vi "UART Read Byte Array.vi"(8 "Error In":errorcluster, 9 "Num Bytes":u8, 10 "UART Channel (0)":u8, 11 "LINX Resource":T1) -> (0 "Error Out":errorcluster, 2 "Data":u8[](array[numeric]), 3 "LINX Resource":T1)   [LabVIEW 2014, in "LMH-LINX.lvlib"]
doc: "Read the specified number of bytes from the specified UART channel's receive buffer as a byte array."
uses:
  LMH-LINX.lvlib
  Private/Type Defs/LINX Ref.ctl
  Private/Type Defs/Platform.ctl
  Private/Type Defs/Interface.ctl
  Private/Device/Type Defs/LINX Device Config.ctl
  Private/Device/Type Defs/TCP Config.ctl
  Private/Device/Type Defs/Channels.ctl
  Private/Type Defs/Peripheral.ctl
  Private/Type Defs/Channel FGV States.ctl
  Private/Device/Device.lvlib
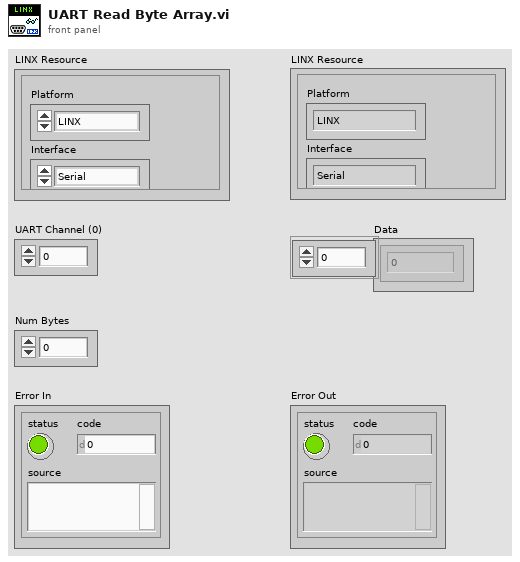
[diagram p1: front panel]
types:
  T1 = typedef "LMH-LINX.lvlib/LINX Ref.ctl" = cluster{"Platform":T2, "Interface":T3, "LINX Device Config":T4}
  T2 = typedef "LMH-LINX.lvlib/Platform.ctl" = enum16{"LINX", "myRIO"}
  T3 = typedef "LMH-LINX.lvlib/Interface.ctl" = enum16{"Serial", "TCP"}
  T4 = typedef "LMH-LINX.lvlib/Device.lvlib/LINX Device Config.ctl" = cluster{"Interface":T3, "COM Port":refnum<visa-resource-name>, "TCP Configuration":T5, "Device Family":u8, "Device ID":u8, "Device Name":string, "TCP Ref":refnum<k5>, "Channels":T6}
  T5 = typedef "LMH-LINX.lvlib/Device.lvlib/TCP Config.ctl" = cluster{"IP Address":string, "Port":u16}
  T6 = typedef "LMH-LINX.lvlib/Channels.ctl" = cluster{"DI":u8[], "DO":u8[], "AI":u8[], "AO":u8[], "PWM":u8[], "QE":u8[], "UART":u8[], "I2C 2":u8[], "SPI":u8[], "CAN":u8[], "Servo":u8[], "AI Ref (V)":dbl, "AO Ref (V)":dbl, "AO Resolution (Bits)":u8}
  T7 = typedef "LMH-LINX.lvlib/Peripheral.ctl" = enum8{"DI", "DO", "AI", "AO", "PWM", "QE", "UART", "I2C", "SPI", "CAN", "Servo"}
  T8 = typedef "LMH-LINX.lvlib/Channel FGV States.ctl" = enum16{"Initialize", "Get", "Set"}
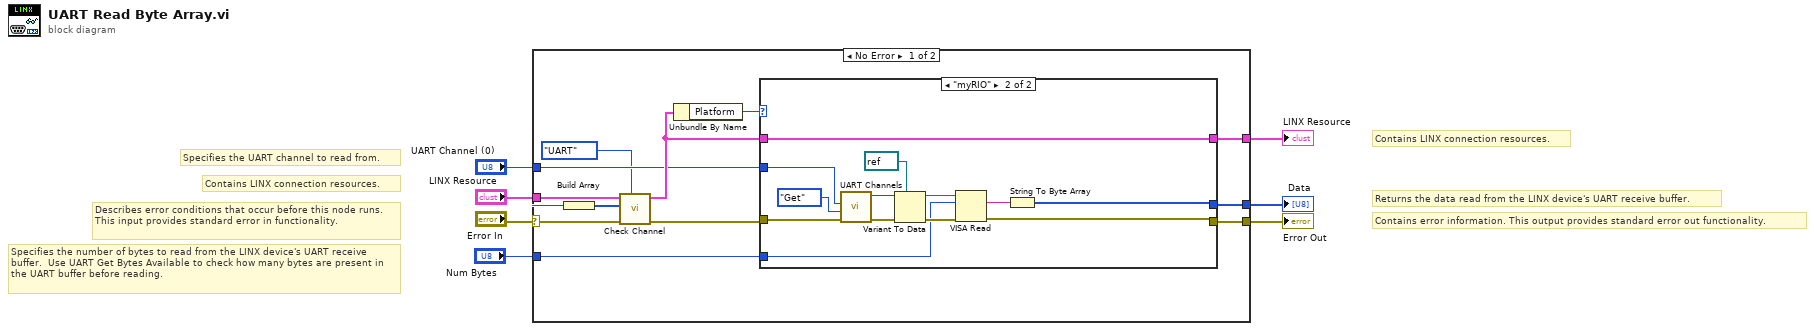
[diagram p0: block diagram]
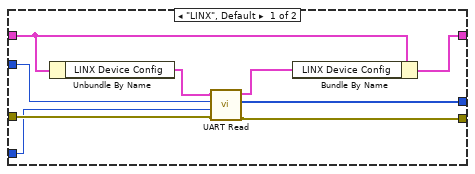
[diagram p2: hidden frame]
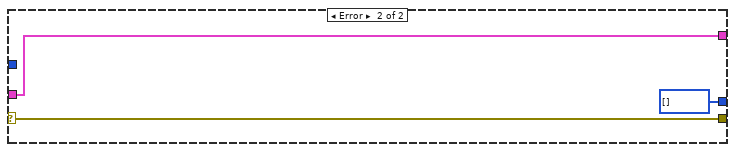
[diagram p3: hidden frame]
diagram:
  # "Specifies the number of bytes to read from the LINX device's UART receive buffer.  Use UART Get Bytes Available to check how many bytes are present in the UART buffer before reading."
  # "Specifies the UART channel to read from."
  # "Returns the data read from the LINX device's UART receive buffer."
  # "Contains LINX connection resources."
  # "Contains error information. This output provides standard error out functionality."
  # "Contains LINX connection resources."
  # "Describes error conditions that occur before this node runs. This input provides standard error in functionality."
  n1 = case shown="No Error" "Error In" {
    selector: "Error In" -> [w8 w44]
    tunnel: [w18 w44] -> w7
    tunnel: [w17 w43] -> w6
    tunnel: "LINX Resource" -> [w16 w43]
    tunnel: "UART Channel (0)" -> [w12 _]
    tunnel: "Num Bytes" -> [w10 _]
    tunnel: [w9 u8[] [] ("unsigned byte array")] -> w2
    frame No Error {
      n2 = Build Array(w12) -> (w13:u8[])
      n3 = call "Check Channel.vi"("Peripheral"=Peripheral."UART", "Error In"=w8, "Channels"=w13, "LINX Resource"=w16) -> ("Error Out"=w14:errorcluster, "LINX Resource"=w15:T1)  [unwired: 5 in, 1 out]
      n4 = Unbundle By Name(w15) -> ("Platform"=w19:T2)
      n5 = case shown="\"myRIO\"" w19 {
        tunnel: w14 -> [w25 w40]
        tunnel: w15 -> [w28 w41]
        tunnel: [w26 w32] -> w18
        tunnel: [w27 w41] -> w17
        tunnel: w12 -> [w21 w36]
        tunnel: [w22 w29] -> w9
        tunnel: w10 -> [w20 w31]
        frame "LINX", Default {
          n6 = Unbundle By Name(w28) -> ("LINX Device Config"=w24:T4)
          n7 = call "UART Read.vi"("Error In"=w25, "Num Bytes"=w20, "UART Channel"=w21, "LINX Device Config"=w24) -> ("Error Out"=w26:errorcluster, "Data"=w22:u8[], "LINX Device Config"=w23:T4)  [unwired: 5 in]
          n8 = Bundle By Name(cluster=w28, "LINX Device Config"=w23) -> (w27:T1)
        }
        frame "myRIO" {
          n9 = call "UART Channels.vi"("Error In"=w40, "Channel State"=Channel_FGV_States."Get", "Channel Number"=w36) -> ("Error Out"=w39:errorcluster, "UART Channel"=w38:variant)  [unwired: 7 in]
          n10 = Variant To Data(error in=w39, type=refnum<visa-resource-name> refnum ("reference"), Variant=w38) -> (data=w34:refnum<visa-resource-name>, error out=w33:errorcluster)
          n11 = VISA Read(VISA resource name=w34, byte count=w31, error in (no error)=w33) -> (read buffer=w30:string, error out=w32:errorcluster)  [unwired: 2 out]
          n12 = String To Byte Array(string=w30) -> (unsigned byte array=w29:u8[])
        }
      }
    }
    frame Error {
    }
  }
  "Error Out" <- w7
  "LINX Resource" <- w6
  "Data" <- w2
